vi "Find Compatible Hardware for Function.vi"(8 "error in (no error)":errorcluster, 10 "Function Name":string, 11 "Controller in":refnum<class "Controller.lvclass">) -> (0 "error out":errorcluster, 3 "Controller out":refnum<class "Controller.lvclass">)   [LabVIEW 2016, in "Controller Actor.lvlib" / "Controller.lvclass"]
uses:
  <userlib>/Common Components/Controller/Controller.lvclass
  C:/Program Files (x86)/National Instruments/LabVIEW 2016/vi.lib/ActorFramework/Actor/Actor.lvclass
  <vilib>/ActorFramework/Actor/Actor.lvclass/Actor.ctl
  <vilib>/ActorFramework/Message Enqueuer/Message Enqueuer.lvclass/Message Enqueuer.ctl
  <userlib>/Common Components/Controller/Messages/Find Devices of Specified Type Msg/Find Devices of Specified Type Msg.lvclass/Find Devices of Specified Type Msg.ctl
  <vilib>/ActorFramework/Message Enqueuer/Init from Existing Queue.vi
  <vilib>/ActorFramework/Message Enqueuer/Enqueue.vi
  <userlib>/Common Components/Controller/Messages/Find Devices of Specified Type Msg/Find Devices of Specified Type Msg.lvclass
  C:/Program Files (x86)/National Instruments/LabVIEW 2016/vi.lib/ActorFramework/Message/Message.lvclass
  <vilib>/ActorFramework/Message Priority Queue/Priority Enqueue.vi
  <vilib>/ActorFramework/Message Enqueuer/Message Enqueuer.lvclass
  <userlib>/Common Components/Function Actor/Function.lvclass
  <vilib>/ActorFramework/Actor/Actor.lvclass
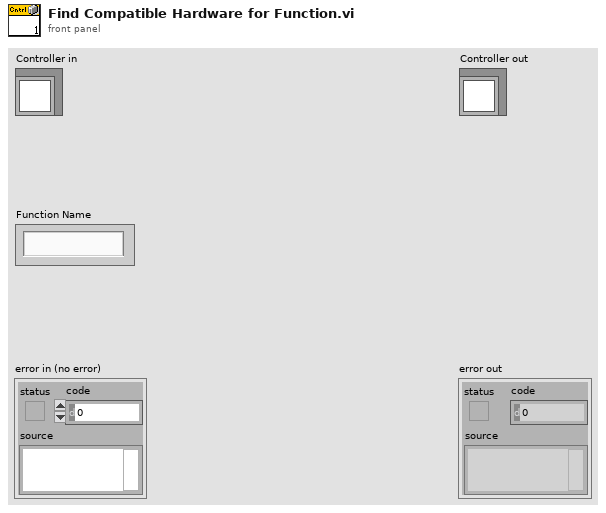
[diagram p1: front panel]
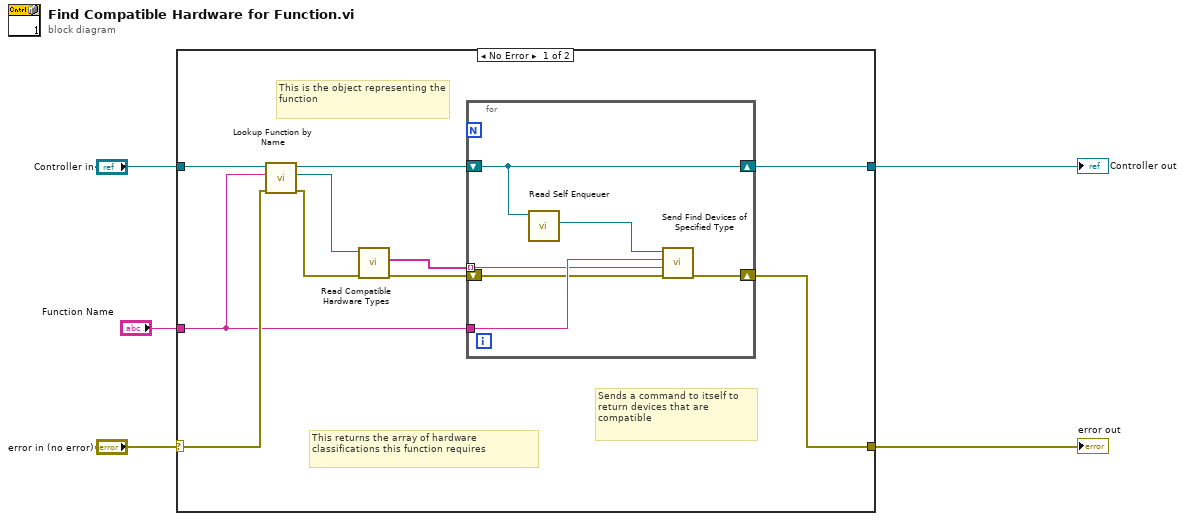
[diagram p0: block diagram]
diagram:
  n1 = case shown="No Error" "error in (no error)" {
    selector: "error in (no error)" -> [w8 w22]
    tunnel: [w7 w22] -> w4
    tunnel: [w11 w21] -> w1
    tunnel: "Controller in" -> [w15 w21]
    tunnel: "Function Name" -> [w6 _]
    frame No Error {
      # "Sends a command to itself to return devices that are compatible"
      # "This returns the array of hardware classifications this function requires"
      # "This is the object representing the function"
      n2 = call <userlib>:"Lookup Function by Name.vi"("error in (no error)"=w8, "Function Name"=w6, "Controller in"=w15) -> ("error out"=w9:errorcluster, "Function.lvclass"=w14:refnum<class "Function.lvclass">, "Controller out"=w13:refnum<class "Controller.lvclass">)  [unwired: 5 in, 1 out]
      n3 = call-dynamic "Read Compatible Hardware Types.vi"("error in (no error)"=w9, "Function in"=w14) -> ("error out"=w10:errorcluster, "Compatible Hardware Types"=w12:string[])  [unwired: 7 in, 1 out]
      n4 = for {
        tunnel: w12 -> [w19] mode=indexing
        shift-right: [w18] -> w11
        shift-left: w13 -> [w18]
        shift-right: [w16] -> w7
        shift-left: w10 -> [w16]
        tunnel: w6 -> [w20]
        n5 = call <vilib>:"Read Self Enqueuer.vi"("Actor"=w18) -> ("Self Enqueuer"=w17:refnum<class "Message Enqueuer.lvclass">)  [unwired: 10 in]
        n6 = call <userlib>:"Send Find Devices of Specified Type.vi"("error in (no error)"=w16, "Hardware Type"=w19, "Function Name"=w20, "Message Enqueuer"=w17) -> ()  [unwired: 6 in, 2 out]
      }
    }
    frame Error {
    }
  }
  "error out" <- w4
  "Controller out" <- w1
